vi "Realsense Cam Reconnect.vi"(8 "error in (no error)":errorcluster, 11 "Realsense Cam in":refnum<class "Realsense Cam.lvclass">) -> (0 "error out":errorcluster, 1 "init error":string, 2 "Found?":bool, 3 "Realsense Cam out":refnum<class "Realsense Cam.lvclass">)   [LabVIEW 2018, in "Realsense Cam.lvclass"]
uses:
  Realsense Cam.lvclass
  Realsense Cam.lvclass/Realsense Cam.ctl
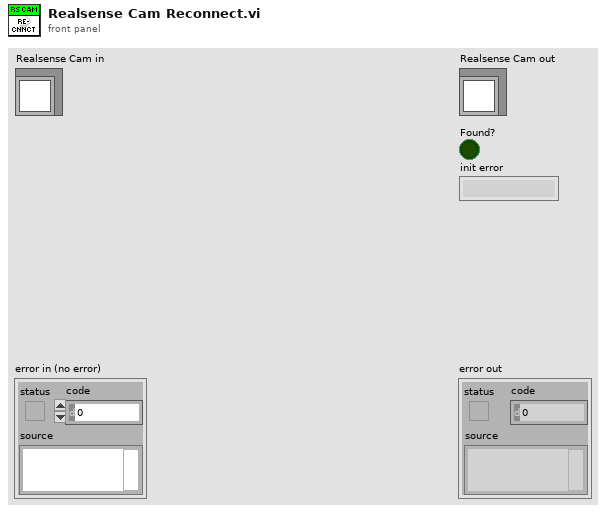
[diagram p1: front panel]
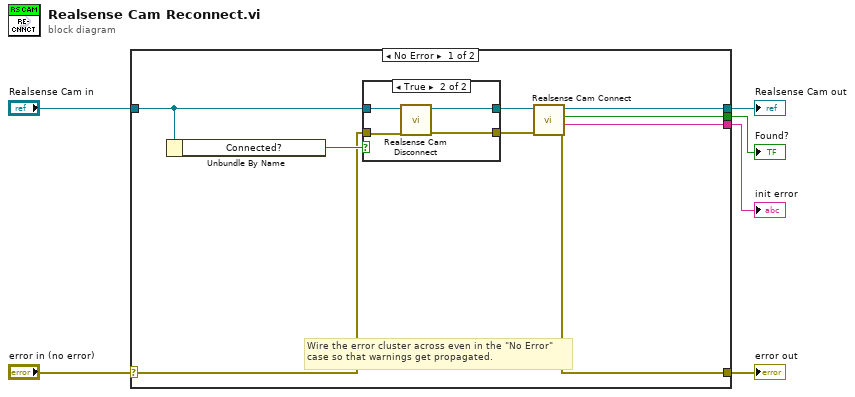
[diagram p0: block diagram]
diagram:
  n1 = case shown="No Error" "error in (no error)" {
    selector: "error in (no error)" -> [w11 w23]
    tunnel: [w9 w23] -> w5
    tunnel: [w15 w22] -> w3
    tunnel: "Realsense Cam in" -> [w13 w22]
    tunnel: [w8 _] -> w2
    tunnel: [w7 _] -> w1
    frame No Error {
      # "Wire the error cluster across even in the \"No Error\"\ncase so that warnings get propagated."
      n2 = Unbundle By Name(w13) -> ("Connected?"=w12:bool)
      n3 = case shown="True" w12 {
        tunnel: w13 -> [w17 w21]
        tunnel: [w17 w20] -> w14
        tunnel: w11 -> [w16 w19]
        tunnel: [w16 w18] -> w10
        frame False {
        }
        frame True {
          n4 = call-dynamic "Realsense Cam Disconnect.vi"("error in (no error)"=w19, "Realsense Cam in"=w21) -> ("error out"=w18:errorcluster, "Realsense Cam out"=w20:refnum<class "Realsense Cam.lvclass">)  [unwired: 7 in, 1 out]
        }
      }
      n5 = call-dynamic "Realsense Cam Connect.vi"("error in (no error)"=w10, "Realsense Cam In"=w14) -> ("error out"=w9:errorcluster, "init error"=w7:string, "Found?"=w8:bool, "Realsense Cam Out"=w15:refnum<class "Realsense Cam.lvclass">)  [unwired: 6 in]
    }
    frame Error {
    }
  }
  "error out" <- w5
  "Realsense Cam out" <- w3
  "Found?" <- w2
  "init error" <- w1
